vi "TAG SubVI.vi"(0 "TAG String":string) -> (1 "TAG":u8[](array[numeric]), 2 "Length":i32)   [LabVIEW 2012]
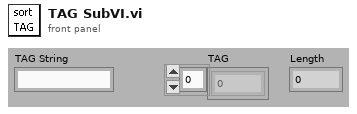
[diagram p1: front panel]
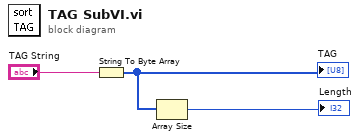
[diagram p0: block diagram]
diagram:
  n1 = String To Byte Array(string="TAG String") -> (unsigned byte array=w2:u8[])
  "TAG" <- w2
  n2 = Array Size(array=w2) -> (size(s)=→"Length":i32)
